vi "FileFreeSpace.vi"(8 "error in (no error)":errorcluster, 11 "controller in":refnum<k24>) -> (0 "error out":errorcluster, 2 "FreeSpace":i32, 3 "controller out":refnum<k24>)   [LabVIEW 2010]
uses:
  c:/aerotech/controller/5.xx.xxx/ensemble/pc/labview/2010/bin/Aerotech.Ensemble.dll
  bin/Aerotech.Ensemble.dll
  c:/aerotech/controller/5.xx.xxx/ensemble/pc/labview/2010/bin/Aerotech.Ensemble.LabVIEW.dll
  bin/Aerotech.Ensemble.LabVIEW.dll
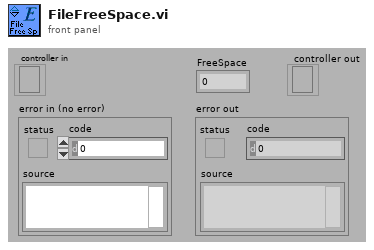
[diagram p1: front panel]
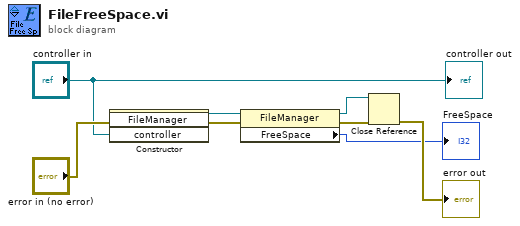
[diagram p0: block diagram]
diagram:
  n1 = constructor class="FileManager"(error in="error in (no error)", "controller"="controller in") -> (reference out=w2:refnum<k24>, error out=w1:errorcluster)  [unwired: 2 in, 2 out]
  n2 = property class="FileManager"(reference=w2, error in=w1) -> (reference out=w7:refnum<k24>, error out=w8:errorcluster, "FreeSpace"=→"FreeSpace":i32)
  n3 = Close Reference(reference=w7, error in (no error)=w8) -> (error out=→"error out":errorcluster)
  "controller out" <- "controller in"
